vi "Test - system-serialization.vi"() -> ()   [LabVIEW 2020]
uses:
  test-device/test-device.lvclass
  test-channel/test-channel.lvclass
  test-group/test-group.lvclass
  test-system/test-system.lvclass
  channel-child/channel-child.lvclass
  C:/code/JKI-JSON-Object-Serialization/JSON Object Serialization/Tests/system-serialization/test-channel/test-channel.lvclass
  <vilib>/addons/_JKI Toolkits/Caraya/classes/Assert/Assert Equal Value_Variant.vi
  <vilib>/addons/_JKI Toolkits/Caraya/classes/Assert/Assert Not Error.vi
  <vilib>/addons/_JKI Toolkits/Caraya/classes/Test/Test.lvclass
  <vilib>/addons/_JKI Toolkits/Caraya/classes/Assert/Assert.lvclass
  test-group-legacy/ test-group-legacy.lvclass
  <vilib>/addons/_JKI Toolkits/Caraya/classes/Assert/Assert True.vi
panel:
  out "result string":string
  out "Unflatten Error":errorcluster
  out "Fake Group String":string
  out "lagacy group class":string
  out "current group class":string
  out "Current Group String":string
  out "legacy Group String":string
  out "flattened system":string
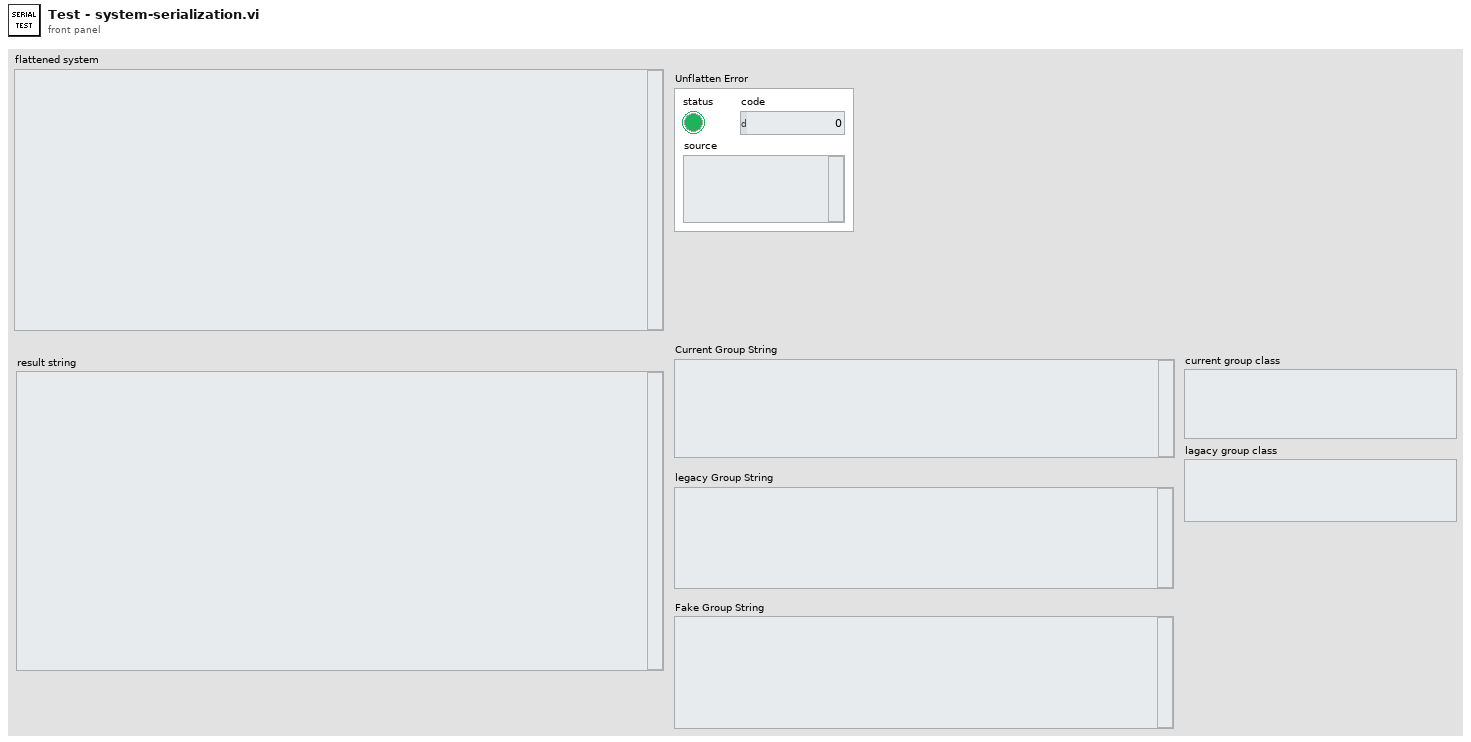
[diagram p1: front panel]
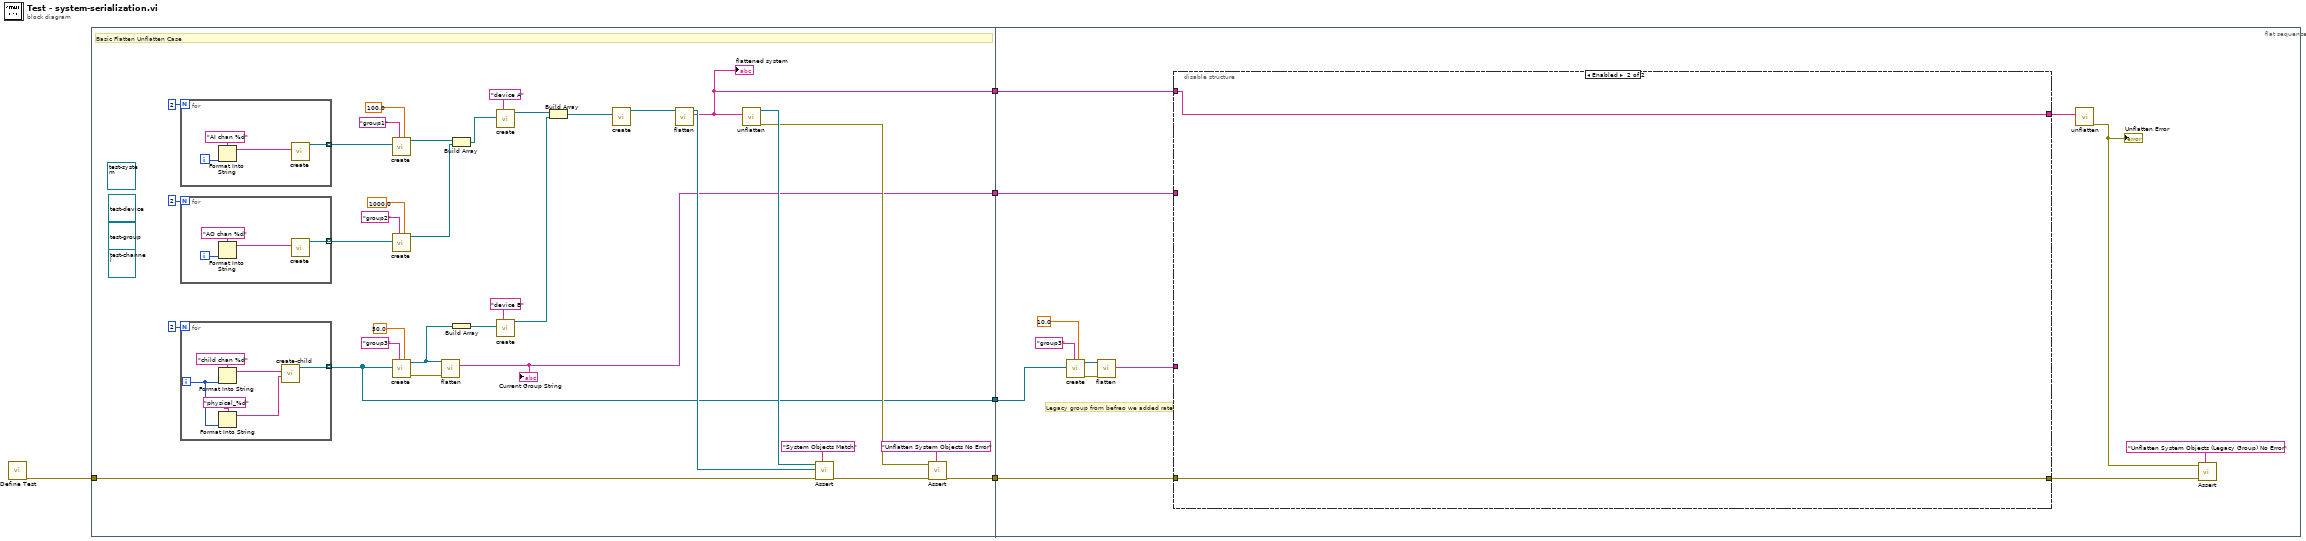
[diagram p0: block diagram]
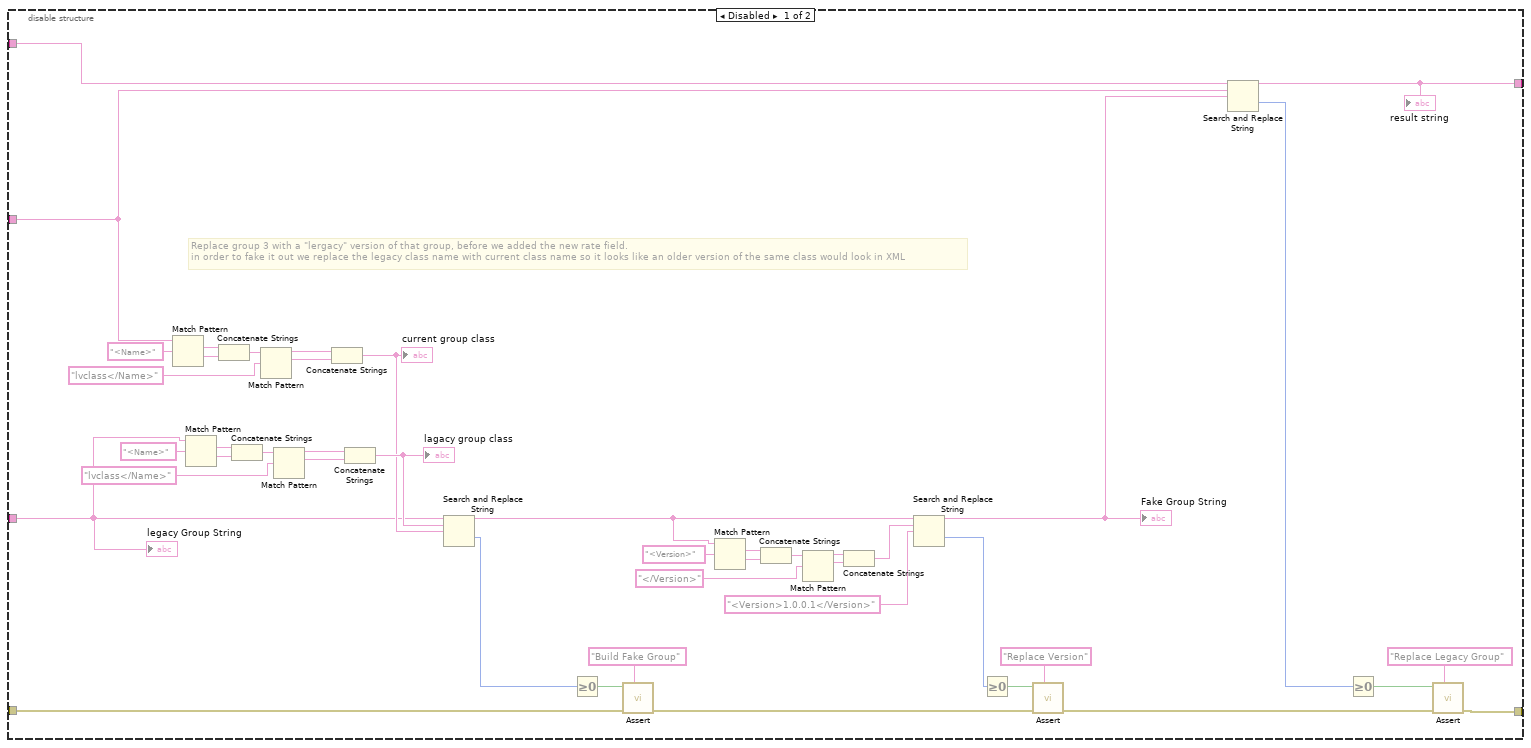
[diagram p2: hidden frame]
diagram:
  n1 = call <vilib>:"Define Test.vi"() -> ("error out"=w5:errorcluster)  [unwired: 10 in, 1 out]
  n2 = flat-sequence {
    tunnel: w5 -> [w19]
    tunnel: [w12] -> w4
    tunnel: [w14] -> w3
    tunnel: [w7] -> w2
    tunnel: [w6] -> w1
    tunnel: w4 -> [w55]
    tunnel: w3 -> [w63]
    tunnel: w2 -> [w58]
    tunnel: w1 -> [w57]
    frame #0 {
      (unwired) refnum<class "test-system.lvclass"> refnum ("test-system.lvclass")
      (unwired) refnum<class "test-group.lvclass"> refnum ("test-group.lvclass")
      (unwired) refnum<class "test-channel.lvclass"> refnum ("test-channel in")
      (unwired) refnum<class "test-device.lvclass"> refnum ("test-device.lvclass")
      # "Basic Flatten Unflatten Case"
      n3 = for {
        N: 2 -> [_]
        tunnel: [w50] -> w39 mode=indexing
        i -> [w53]
        n4 = Format Into String(format string="AI chan %d", w53) -> (resulting string=w51:string)  [unwired: 2 in, 1 out]
        n5 = call "create.vi"("name"=w51) -> ("test-channel out"=w50:refnum<class "test-channel.lvclass">)  [unwired: 9 in, 1 out]
      }
      n6 = for {
        N: 2 -> [_]
        tunnel: [w46] -> w36 mode=indexing
        i -> [w49]
        n7 = Format Into String(format string="AO chan %d", w49) -> (resulting string=w47:string)  [unwired: 2 in, 1 out]
        n8 = call "create.vi"("name"=w47) -> ("test-channel out"=w46:refnum<class "test-channel.lvclass">)  [unwired: 9 in, 1 out]
      }
      n9 = for {
        N: 2 -> [_]
        tunnel: [w44] -> w6 mode=indexing
        i -> [w42]
        n10 = Format Into String(format string="child chan %d", w42) -> (resulting string=w43:string)  [unwired: 2 in, 1 out]
        n11 = Format Into String(format string="physical_%d", w42) -> (resulting string=w40:string)  [unwired: 2 in, 1 out]
        n12 = call "create-child.vi"("physical channel"=w40, "name"=w43) -> ("channel-child out"=w44:refnum<class "channel-child.lvclass">)  [unwired: 8 in, 1 out]
      }
      n13 = call "create.vi"("rate"=100.0, "name"="group1", "test-channel in"=w39) -> ("test-group out"=w31:refnum<class "test-group.lvclass">)  [unwired: 7 in, 1 out]
      n14 = call "create.vi"("rate"=1000.0, "name"="group2", "test-channel in"=w36) -> ("test-group out"=w30:refnum<class "test-group.lvclass">)  [unwired: 7 in, 1 out]
      n15 = call "create.vi"("rate"=50.0, "name"="group3", "test-channel in"=w6) -> ("error out"=w8:errorcluster, "test-group out"=w9:refnum<class "test-group.lvclass">)  [unwired: 7 in]
      n16 = call "flatten.vi"("error in"=w8, "test-group in"=w9) -> ("flattened group"=w7:string)  [unwired: 7 in, 2 out]
      "Current Group String" <- w7
      n17 = Build Array(w31, w30) -> (w29:refnum<class "test-group.lvclass">[])
      n18 = Build Array(w9) -> (w24:refnum<class "test-group.lvclass">[])
      n19 = call "create.vi"("name"="device A", "groups"=w29) -> ("test-device out"=w15:refnum<class "test-device.lvclass">)  [unwired: 8 in, 1 out]
      n20 = call "create.vi"("name"="device B", "groups"=w24) -> ("test-device out"=w23:refnum<class "test-device.lvclass">)  [unwired: 8 in, 1 out]
      n21 = Build Array(w15, w23) -> (w22:refnum<class "test-device.lvclass">[])
      n22 = call "create.vi"("devices"=w22) -> ("test-system out"=w20:refnum<class "test-system.lvclass">)  [unwired: 9 in, 1 out]
      n23 = call "flatten.vi"("test-system in"=w20) -> ("flattened system"=w14:string, "test-system out"=w17:refnum<class "test-system.lvclass">)  [unwired: 8 in, 1 out]
      "flattened system" <- w14
      n24 = call "unflatten.vi"("flattened system"=w14) -> ("error out"=w11:errorcluster, "test-system out"=w18:refnum<class "test-system.lvclass">)  [unwired: 9 in]
      n25 = call-poly <vilib>:"Assert.vi"("Label"="System Objects Match", "error in (no error)"=w19, "Y"=w17, "X"=w18) -> ("error out"=w13:errorcluster)  [unwired: 6 in, 1 out]
      n26 = call-poly <vilib>:"Assert.vi"("Label"="Unflatten System Objects No Error", "error in (no error)"=w13, "Not Error?"=w11) -> ("error out"=w12:errorcluster)  [unwired: 7 in, 1 out]
    }
    frame #1 {
      # "Legacy group from befreo we added rate"
      n27 = call "create.vi"("rate"=10.0, "name"="group3", "test-channel in"=w57) -> ("error out"=w64:errorcluster, "test-group-legacy out"=w65:refnum<class " test-group-legacy.lvclass">)  [unwired: 7 in]
      n28 = call "flatten.vi"("error in"=w64, "test-group-legacy in"=w65) -> ("flattened group"=w54:string)  [unwired: 7 in, 2 out]
      n29 = disable-structure shown="Enabled" {
        disable-tunnel: w63 -> [w109 w110]
        disable-tunnel: [w108 w110] -> w62
        disable-tunnel: [w104 w111] -> w60
        disable-tunnel: w58 -> [w103 _]
        disable-tunnel: w55 -> [w69 w111]
        disable-tunnel: w54 -> [w68 _]
        frame Disabled {
          # "Replace group 3 with a \"lergacy\" version of that group, before we added the new rate field.\nin order to fake it out we replace the legacy class name with current class name so it looks like an older version of the same class would look in XML"
          n30 = Match Pattern(string=w103, regular expression="<Name>") -> (match substring=w101:string, after substring=w100:string)  [unwired: 1 in, 2 out]
          n31 = Match Pattern(string=w68, regular expression="<Name>") -> (match substring=w90:string, after substring=w91:string)  [unwired: 1 in, 2 out]
          n32 = Concatenate Strings(w101, w100) -> (w99:string)
          n33 = Concatenate Strings(w90, w91) -> (w92:string)
          n34 = Match Pattern(string=w99, regular expression="lvclass</Name>") -> (before substring=w96:string, match substring=w97:string)  [unwired: 1 in, 2 out]
          n35 = Match Pattern(string=w92, regular expression="lvclass</Name>") -> (before substring=w95:string, match substring=w94:string)  [unwired: 1 in, 2 out]
          n36 = Concatenate Strings(w96, w97) -> (w87:string)
          "current group class" <- w87
          n37 = Concatenate Strings(w95, w94) -> (w88:string)
          "lagacy group class" <- w88
          n38 = Search and Replace String(input string=w68, search string=w88, replace string=w87) -> (result string=w67:string, offset past replacement=w84:i32)  [unwired: 5 in, 2 out]
          n39 = Greater Or Equal To 0?(x=w84) -> (x >= 0?=w85:bool)
          n40 = call-poly <vilib>:"Assert.vi"("Label"="Build Fake Group", "error in (no error)"=w69, "True?"=w85) -> ("error out"=w83:errorcluster)  [unwired: 7 in, 1 out]
          n41 = Match Pattern(string=w67, regular expression="<Version>") -> (match substring=w81:string, after substring=w80:string)  [unwired: 1 in, 2 out]
          n42 = Concatenate Strings(w81, w80) -> (w79:string)
          n43 = Match Pattern(string=w79, regular expression="</Version>") -> (before substring=w76:string, match substring=w77:string)  [unwired: 1 in, 2 out]
          n44 = Concatenate Strings(w76, w77) -> (w75:string)
          n45 = Search and Replace String(input string=w67, search string=w75, replace string="<Version>1.0.0.1</Version>" ("regular expression")) -> (result string=w70:string, offset past replacement=w71:i32)  [unwired: 5 in, 2 out]
          "Fake Group String" <- w70
          n46 = Greater Or Equal To 0?(x=w71) -> (x >= 0?=w73:bool)
          n47 = call-poly <vilib>:"Assert.vi"("Label"="Replace Version", "True?"=w73) -> ()  [unwired: 8 in, 2 out]
          n48 = Search and Replace String(input string=w109, search string=w103, replace string=w70) -> (result string=w108:string, offset past replacement=w107:i32)  [unwired: 5 in, 2 out]
          "result string" <- w108
          n49 = Greater Or Equal To 0?(x=w107) -> (x >= 0?=w106:bool)
          n50 = call-poly <vilib>:"Assert.vi"("Label"="Replace Legacy Group", "error in (no error)"=w83, "True?"=w106) -> ("error out"=w104:errorcluster)  [unwired: 7 in, 1 out]
          "legacy Group String" <- w68
        }
        frame Enabled {
        }
      }
      n51 = call "unflatten.vi"("flattened system"=w62) -> ("error out"=w59:errorcluster)  [unwired: 9 in, 1 out]
      "Unflatten Error" <- w59
      n52 = call-poly <vilib>:"Assert.vi"("Label"="Unflatten System Objects (Legacy Group) No Error", "error in (no error)"=w60, "Not Error?"=w59) -> ()  [unwired: 7 in, 2 out]
    }
  }
